vi "3HeActualPressure.vi"(11 "3He Pressure (Torr)":string="1") -> (0 "Actual 3He\nTank Pressure":dbl min=0.0 max=100.0 step=5.0 format="%#.1g")   [LabVIEW 2018]
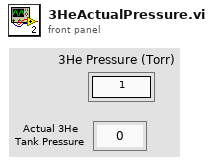
[diagram p1: front panel]
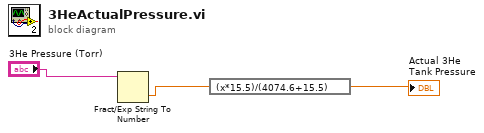
[diagram p0: block diagram]
diagram:
  n1 = Fract/Exp String To Number(string="3He Pressure (Torr)") -> (number=w2:dbl)  [unwired: 3 in, 1 out]
  n2 = expression code="(x*15.5)/(4074.6+15.5)"(w2) -> (→"Actual 3He\nTank Pressure":dbl)
